vi "microspectrometer_standalone.vi"() -> ()   [LabVIEW 2013]
uses:
  <vilib>/Instr/_visa.llb/VISA Configure Serial Port (Instr).vi
panel:
  in  "intergation time":dbl=54.0 min=54.0 max=5000000.0 step=100.0
  out "XY-Graph 3":cluster{i32[], u16[]}(graph) caption="sensor signal"
  in  "pause measure":bool
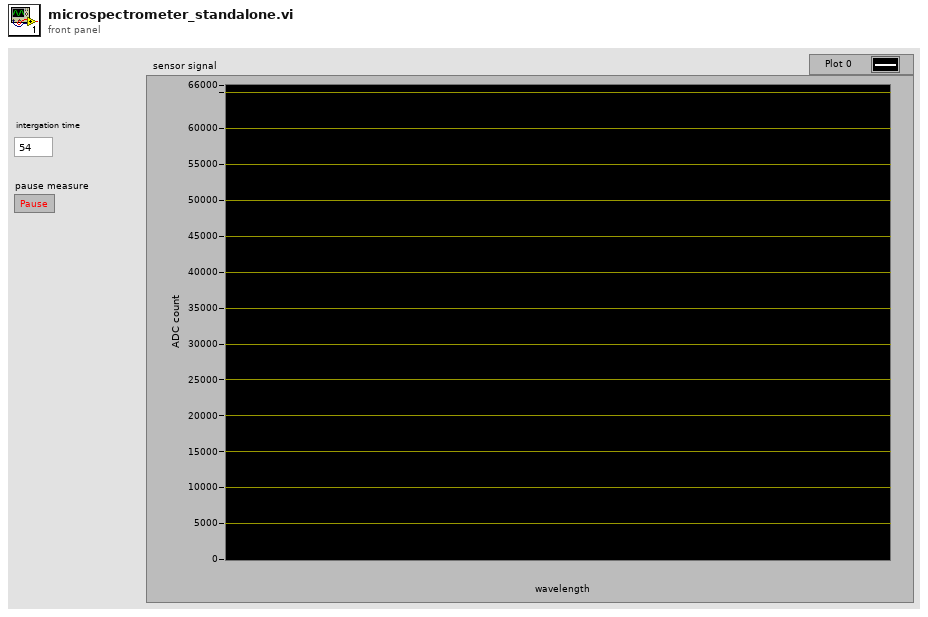
[diagram p1: front panel]
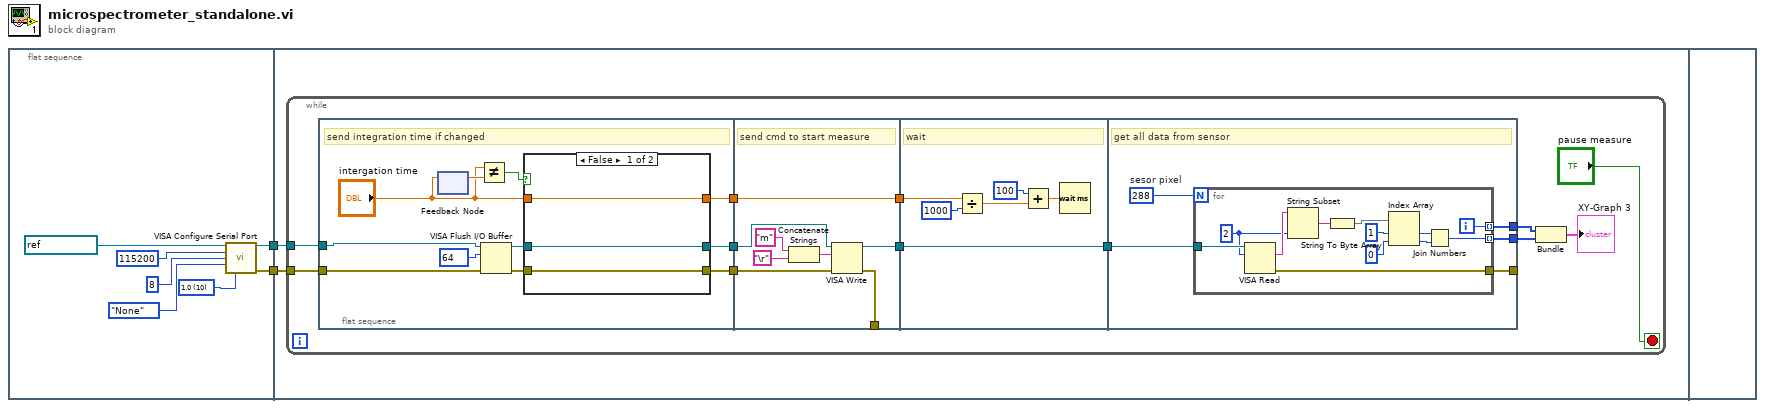
[diagram p0: block diagram]
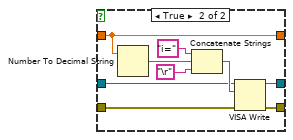
[diagram p2: hidden frame]
diagram:
  n1 = flat-sequence {
    tunnel: [w5] -> w2
    tunnel: [w4] -> w1
    tunnel: w2 -> [w11]
    tunnel: w1 -> [w10]
    frame #0 {
      w6 = u16 10 items=["1.0"=10, "1.5"=15, "2.0"=20] ("stop bits (10: 1 bit)")
      n2 = call-poly "VISA Configure Serial Port"("VISA resource name"=refnum<visa-resource-name> "COM11", "baud rate (9600)"=u32 115200, "data bits (8)"=u16 8, "parity (0:none)"=enum16{"None", "Odd", "Even", "Mark", "Space"}."None", "stop bits (10: 1 bit)"=w6) -> ("VISA resource name out"=w5:refnum<visa-resource-name>, "error out"=w4:errorcluster)  [unwired: 9 in]
    }
    frame #1 {
      n3 = while {
        tunnel: w11 -> [w21]
        tunnel: w10 -> [w20]
        stop <- "pause measure" stop-if-true
        n4 = flat-sequence {
          tunnel: w21 -> [w33]
          tunnel: w20 -> [w34]
          tunnel: [w28] -> w18
          tunnel: [w27] -> w17
          tunnel: [w25] -> w16
          tunnel: [w51] -> w22
          tunnel: [w50] -> _
          tunnel: w18 -> [w48]
          tunnel: w17 -> [w49]
          tunnel: w16 -> [w47]
          tunnel: [w47] -> w15
          tunnel: w22 -> [w56]
          tunnel: [w56] -> w19
          tunnel: w15 -> [w55]
          tunnel: w19 -> [w64]
          tunnel: [w65] -> _
          tunnel: [w63] -> w13
          tunnel: [w62] -> w12
          frame #0 {
            # "send integration time if changed"
            n5 = feedback #1() -> (w32:dbl)  [unwired: 1 in]
            n6 = feedback-in #1("intergation time") -> ()
            n7 = Not Equal?(x="intergation time", y=w32) -> (x != y?=w31:bool)
            n8 = VISA Flush I/O Buffer(VISA resource name=w33, mask (16)=64, error in (no error)=w34) -> (VISA resource name out=w30:refnum<visa-resource-name>, error out=w29:errorcluster)
            n9 = case shown="False" w31 {
              tunnel: w30 -> [w36 w42]
              tunnel: w29 -> [w35 w41]
              tunnel: [w35 w40] -> w28
              tunnel: [w36 w39] -> w27
              tunnel: "intergation time" -> [w37 w38]
              tunnel: [w37 w38] -> w25
              frame False {
              }
              frame True {
                n10 = Number To Decimal String(number=w38) -> (decimal integer string=w45:string)  [unwired: 1 in]
                n11 = Concatenate Strings("i=", w45, "\r") -> (w43:string)
                n12 = VISA Write(VISA resource name=w42, write buffer=w43, error in (no error)=w41) -> (VISA resource name out=w39:refnum<visa-resource-name>, error out=w40:errorcluster)  [unwired: 1 out]
              }
            }
          }
          frame #1 {
            # "send cmd to start measure"
            n13 = Concatenate Strings("m", "\r") -> (w52:string)
            n14 = VISA Write(VISA resource name=w49, write buffer=w52, error in (no error)=w48) -> (VISA resource name out=w51:refnum<visa-resource-name>, error out=w50:errorcluster)  [unwired: 1 out]
          }
          frame #2 {
            # "wait"
            n15 = Divide(x=w55, y=u32 1000 ("Zu wartende ms")) -> (x/y=w57:dbl)
            n16 = Add(x=u32 100 ("Zu wartende ms"), y=w57) -> (x+y=w59:dbl)
            n17 = Wait (ms)(milliseconds to wait=w59) -> ()  [unwired: 1 out]
          }
          frame #3 {
            w61 = 288  # sesor pixel
            # "get all data from sensor"
            n18 = for {
              N: w61 -> [_]
              tunnel: w64 -> [w77]
              tunnel: [w68] -> w65
              tunnel: [w67] -> w63 mode=indexing
              tunnel: [w66] -> w62 mode=indexing
              i -> [w66]
              w75 = 2
              n19 = VISA Read(VISA resource name=w77, byte count=w75) -> (read buffer=w76:string, error out=w68:errorcluster)  [unwired: 1 in, 2 out]
              n20 = String Subset(string=w76, length (rest)=w75) -> (substring=w74:string)  [unwired: 1 in]
              n21 = String To Byte Array(string=w74) -> (unsigned byte array=w73:u8[])
              n22 = Index Array(array=w73, index #1=1, index #2=0) -> (element #1=w69:u8, element #2=w70:u8)
              n23 = Join Numbers(hi=w69, lo=w70) -> ((hi.lo)=w67:u16)
            }
          }
        }
        n24 = Bundle(w12, w13) -> (→"XY-Graph 3":cluster{i32[], u16[]})  [unwired: 1 in]
      }
    }
    frame #2 {
    }
  }
